vi "Configure test.vi"(6 "Assert VI Path":path, 7 "Existing Queue Elements":string, 8 "error in (no error)":errorcluster, 11 "Basic Boolean in":refnum<class "Boolean.lvclass">) -> (0 "error out":errorcluster)   [LabVIEW 2018, in "Boolean.lvclass"]
uses:
  Boolean.lvclass
  Test.lvclass
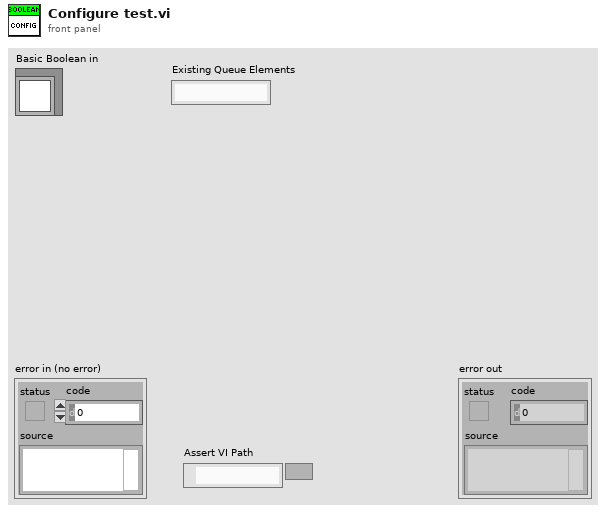
[diagram p1: front panel]
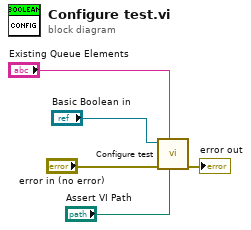
[diagram p0: block diagram]
diagram:
  n1 = call-parent "Configure test.vi"("Assert VI Path"="Assert VI Path", "Existing Queue Elements"="Existing Queue Elements", "error in (no error)"="error in (no error)", "Basic Test in"="Basic Boolean in") -> ("error out"=→"error out":errorcluster)  [unwired: 7 in]
